vi "To Service.vi"(11 "Entity Manager":refnum<class "Entity Manager.lvclass">) -> (3 "Entity Manager Service":refnum<class "Entity Manager Service.lvclass">)   [LabVIEW 2022 SP3, in "HTTP-Conditum.lvlib" / "Entity Manager Service.lvclass"]
uses:
  Entity Manager Service.lvclass
  Entity Manager Service.lvclass/Entity Manager Service.ctl
  <vilib>/IlluminatedG/IG Conditum/Conditum/Entity Manager/Entity Manager.lvclass
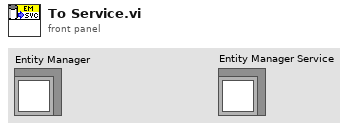
[diagram p1: front panel]
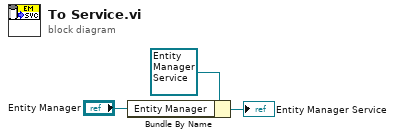
[diagram p0: block diagram]
diagram:
  n1 = Bundle By Name(cluster=refnum<class "Entity Manager Service.lvclass"> refnum ("Entity Manager Service out"), "Entity Manager"="Entity Manager") -> (→"Entity Manager Service":refnum<class "Entity Manager Service.lvclass">)
